vi "Get Item.vi"(8 "error in (no error)":errorcluster, 10 "Tag Name":string, 11 "Current Value Table in":refnum<class "Current Value Table.lvclass">) -> (0 "error out":errorcluster, 2 "CVT_Item out":refnum<class "iCVT_Item.lvclass">, 3 "Current Value Table out":refnum<class "Current Value Table.lvclass">)   [LabVIEW 2024, in "Current Value Table.lvlib" / "Current Value Table.lvclass"]
uses:
  Current Value Table.lvclass
  iCVT_Item/iCVT_Item.lvclass
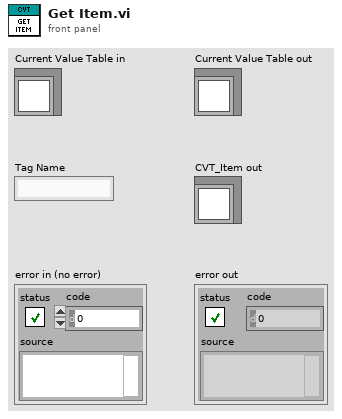
[diagram p1: front panel]
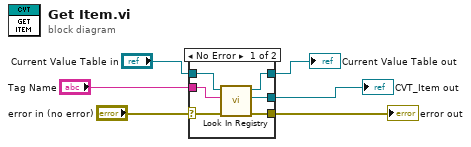
[diagram p0: block diagram]
diagram:
  n1 = case shown="No Error" "error in (no error)" {
    selector: "error in (no error)" -> [w10 w14]
    tunnel: [w7 w14] -> w5
    tunnel: [w8 w13] -> w3
    tunnel: "Current Value Table in" -> [w12 w13]
    tunnel: "Tag Name" -> [w11 _]
    tunnel: [w9 _] -> w1
    frame No Error {
      n2 = call-dynamic "Look In Registry.vi"("error in (no error)"=w10, "Tag Name"=w11, "Current Value Table in"=w12) -> ("error out"=w7:errorcluster, "CVT_Item out"=w9:refnum<class "iCVT_Item.lvclass">, "Current Value Table out"=w8:refnum<class "Current Value Table.lvclass">)  [unwired: 5 in, 1 out]
    }
    frame Error {
    }
  }
  "error out" <- w5
  "Current Value Table out" <- w3
  "CVT_Item out" <- w1
